vi "Stop.vi"(6 "Error":errorcluster, 7 "ConcreteActor":refnum<class "ConcreteActor.lvclass">) -> (4 "Error":errorcluster, 5 "ConcreteActor":refnum<class "ConcreteActor.lvclass">)   [LabVIEW 2020, in "jettl.lvlib" / "Base.lvlib" / "ConcreteActor.lvclass"]
uses:
  ConcreteActor.lvclass
  ConcreteActor.lvclass/ConcreteActor.ctl
  C:/jettl-harness/repos/jettl/src/jettl/jettl/Base/ConcreteActor/ConcreteActor.lvclass
  C:/jettl-harness/repos/jettl/src/jettl/jettl/Actor/Actor.lvclass
  jettl.lvlib
  Lifetime.ctl
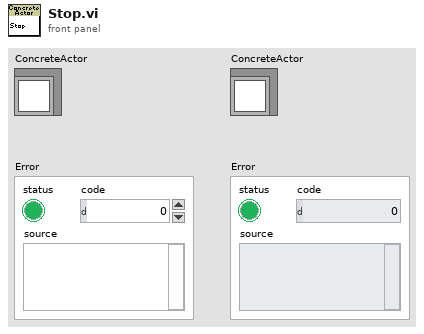
[diagram p1: front panel]
types:
  T1 = typedef "jettl.lvlib/Lifetime.ctl" = enum16{"Setup", "TeardownBeforeStart", "Start", "Running", "Stop", "TeardownAfterStart"}
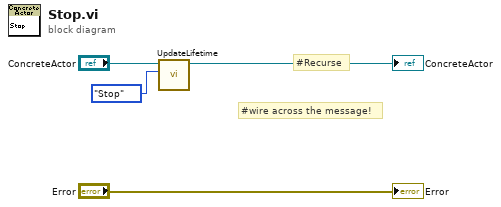
[diagram p0: block diagram]
diagram:
  # "#wire across the message!"
  # "#Recurse"
  n1 = call "UpdateLifetime.vi"("Lifetime"=Lifetime."Stop", "Actor"="ConcreteActor") -> ("Actor"=→"ConcreteActor":refnum<class "ConcreteActor.lvclass">)  [unwired: 9 in]
  "Error" <- "Error"
